vi "Laser 1 TL UI handler L3.vi"(5 "VISA Resource":T2[](array[typedef]), 6 "Numeric":dbl[](array[numeric]), 7 "FP Ops":T4(ring), 8 "Error in":errorcluster caption="Error in (no error)", 9 "Boolean":bool, 10 "I/p string(s)":string[](array[string]), 11 "UI elements cluster":T1) -> (0 "Error out":errorcluster, 3 "Ls1 User Controls 2":T3)   [LabVIEW 2020]
uses:
  Type Defs/Ls1 User Controls.ctl
  Serial Comms/Visa resource.ctl
  Typedefs/Plane Mode.ctl
  Typedefs/Laser control knob.ctl
  Typedefs/PMT control knob.ctl
  Typedefs/XY Stage_Move.ctl
  Typedefs/Frame Size.ctl
  Typedefs/UI ctrl refs cluster.ctl
  Typedefs/test_fpga_control.ctl
  User Interface/Misc/Biology Information.ctl
  User Interface/Misc/Experiment Type.ctl
  Acquisition/Typedefs/Ref DAQ Param.ctl
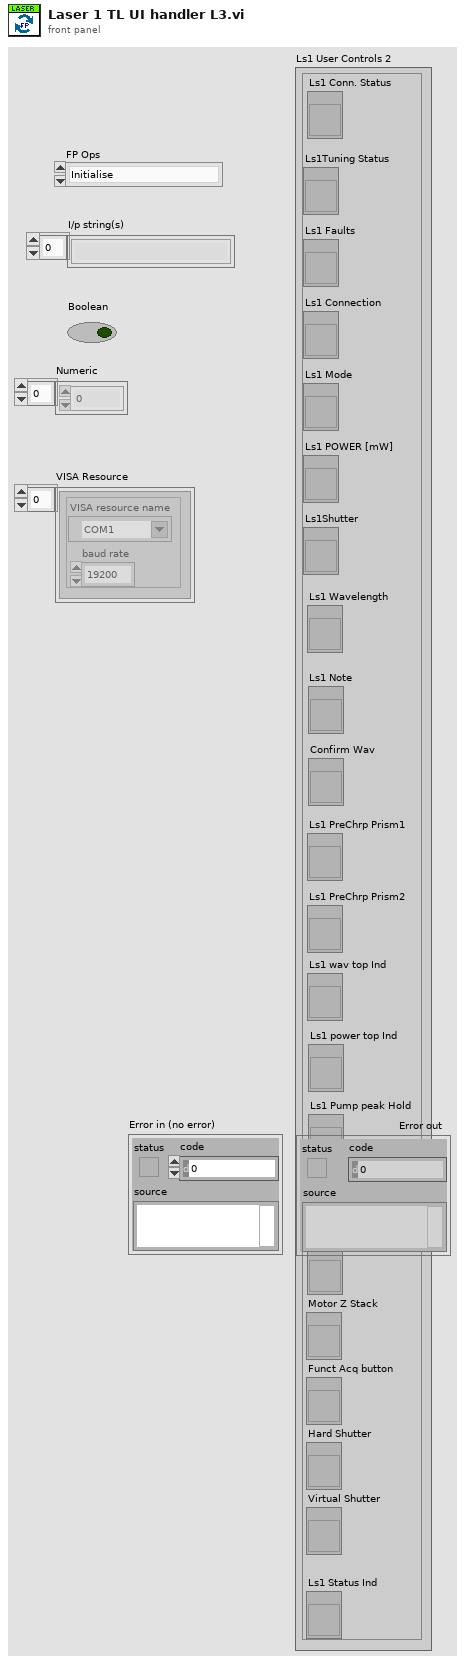
[diagram p1: front panel]
types:
  T1 = typedef "UI ctrl refs cluster.ctl" = cluster{"Top level VI path":path, "Top level VI ref":refnum<vi>, "User menu ref":refnum<k9>, "Sub Panel control":refnum<vi>, "Imaging Param Tab":refnum<vi>, "Occurrence-Start drivers":refnum<k4>, "Occurrence-Speed logging initialised":refnum<k4>, "Occurrence-XYZ stage initialised":refnum<k4>, "Exit button":refnum<vi>, "Status ind":refnum<vi>, "Set as origin":refnum<vi>, "Speed Logging":refnum<vi>, "Time Lapse":refnum<vi>, "Live Imaging":refnum<vi>, "AOL Z Stack":refnum<vi>, "Motor Z Stack":refnum<vi>, "Funct Acq button":refnum<vi>, "Hard Shutter":refnum<vi>, "Virtual Shutter":refnum<vi>, "Laser Power":refnum<vi>, "AOL Mode":refnum<vi>, "Frame Size":refnum<vi>, "Field of View":refnum<vi>, "Dwell Time":refnum<vi>, "Zoom":refnum<vi>, "AOL Z":refnum<vi>, "Objective":refnum<vi>, "Axis":refnum<vi>, "Paths & Names":refnum<vi>, "Experiment folder path (ind.)":refnum<vi>, "Last State (Ind.)":refnum<vi>, "Averages":refnum<vi>, "Angle (degrees)":refnum<vi>, "X centre":refnum<vi>, "Y centre":refnum<vi>, "Plane Mode":refnum<vi>, "# Planes":refnum<vi>, "Z Start":refnum<vi>, "Z Stop":refnum<vi>, "Z Step":refnum<vi>, "PMT 1":refnum<vi>, "PMT 2":refnum<vi>, "Stage XYZ Position":refnum<vi>, "Pockels@Z Start":refnum<vi>, "Pockels@Z Stop":refnum<vi>, "Obtain Z Start":refnum<vi>, "Obtain Z Stop":refnum<vi>, "Live stim.trig.period":refnum<vi>, "Live stim.trig.enable":refnum<vi>, "Movement Correction":refnum<vi>, "Load Reference Image":refnum<vi>, "XY Stage Move":refnum<vi>, "MovCor Cluster":refnum<vi>, "RefDAQParam":refnum<vi>, "Funct. Acq. Pockels Modulation":refnum<vi>, "Ref Laser Power":refnum<vi>, "Enable Video Recording":refnum<vi>, "Video Record-Live Imaging":refnum<vi>, "Video Record-Funct acq":refnum<vi>, "Reference Source":refnum<vi>, "AOL Z-stack Chirps Ready (ind)":refnum<vi>, "Target time between mov.cor. ref triggers (ms)":refnum<vi>, "Funct. Acq. Ref frame save":refnum<vi>, "Tracking button":refnum<vi>, "Show ref plots window":refnum<vi>, "Center freq ind (nm)":refnum<vi>, "Pickup mode (ind)":refnum<vi>, "Logging queue (ind)":refnum<vi>, "Back aperture power (ind.)":refnum<vi>, "Power after objective (ind.)":refnum<vi>, "Switch user":refnum<vi>, "Ls1 Conn. Status":refnum<vi>, "Ls1Tuning Status":refnum<vi>, "Ls1 Faults":refnum<vi>, "Ls1 Connection":refnum<vi>, "Ls1 Mode":refnum<vi>, "Ls1 POWER [mW]":refnum<vi>, "Ls1Shutter":refnum<vi>, "Ls1 Wavelength":refnum<vi>, "Ls1 Note":refnum<vi>, "Ls1 Confirm Wav":refnum<vi>, "Ls1 PreChrp Prism1":refnum<vi>, "Ls1 PreChrp Prism2":refnum<vi>, "Ls1 wav top Ind":refnum<vi>, "Ls1 power top Ind":refnum<vi>, "Ls1 Pump peak Hold":refnum<vi>, "Ls1 Status Ind":refnum<vi>, "Ls1 wav cancel":refnum<vi>, "Experiment Type":refnum<vi>, "Biology Information":refnum<vi>, "Camera recording status":refnum<vi>}
  T2 = typedef "Visa resource.ctl" = cluster{"VISA resource name":refnum<visa-resource-name>, "baud rate":u32}
  T3 = typedef "Ls1 User Controls.ctl" = cluster{"Ls1 Conn. Status":refnum<vi>, "Ls1Tuning Status":refnum<vi>, "Ls1 Faults":refnum<vi>, "Ls1 Connection":refnum<vi>, "Ls1 Mode":refnum<vi>, "Ls1 POWER [mW]":refnum<vi>, "Ls1Shutter":refnum<vi>, "Ls1 Wavelength":refnum<vi>, "Ls1 Note":refnum<vi>, "Confirm Wav":refnum<vi>, "Ls1 PreChrp Prism1":refnum<vi>, "Ls1 PreChrp Prism2":refnum<vi>, "Ls1 wav top Ind":refnum<vi>, "Ls1 power top Ind":refnum<vi>, "Ls1 Pump peak Hold":refnum<vi>, "Live Imaging":refnum<vi>, "AOL Z Stack":refnum<vi>, "Motor Z Stack":refnum<vi>, "Funct Acq button":refnum<vi>, "Hard Shutter":refnum<vi>, "Virtual Shutter":refnum<vi>, "Ls1 Status Ind":refnum<vi>}
  T4 = enum16{"Initialise", "Disable Controls", "Enable Controls", "Update Connection Info", "Update Laser Warning", "Update Laser status", "Update Laser Wav.", "Update prechiper settings", "Update Laser Note", "Update Shutter Status"}
  T5 = enum8{"Enabled", "Disabled", "Disabled and Grayed Out"}
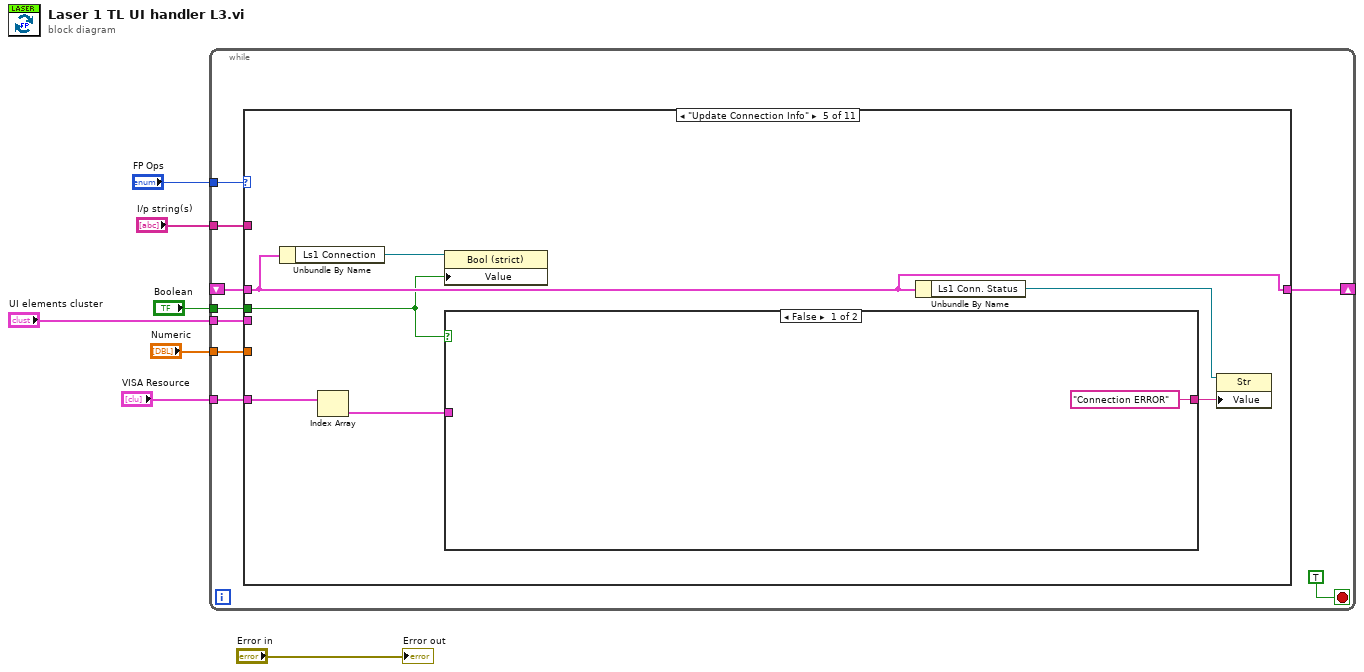
[diagram p0: block diagram]
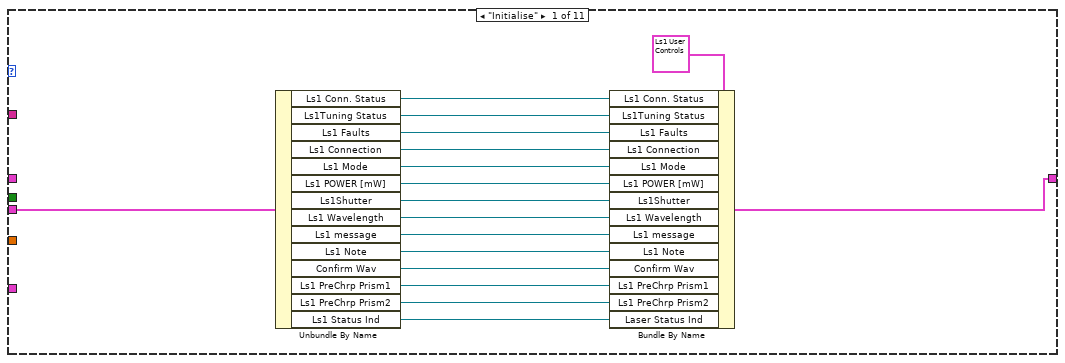
[diagram p2: hidden frame]
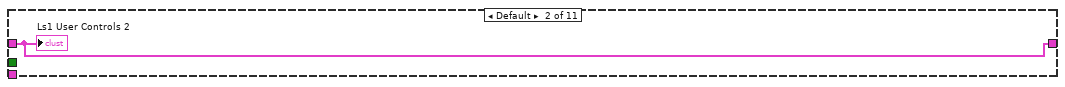
[diagram p3: hidden frame]
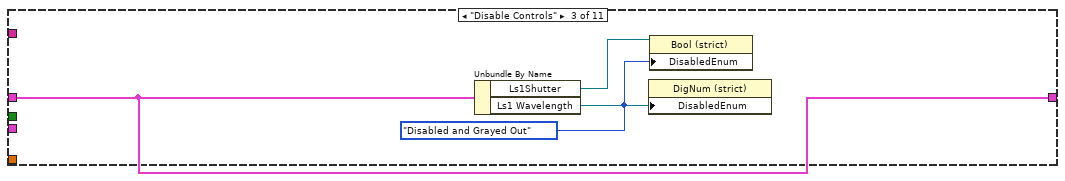
[diagram p4: hidden frame]
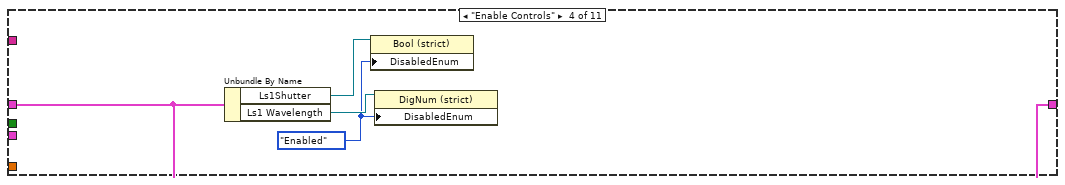
[diagram p5: hidden frame]
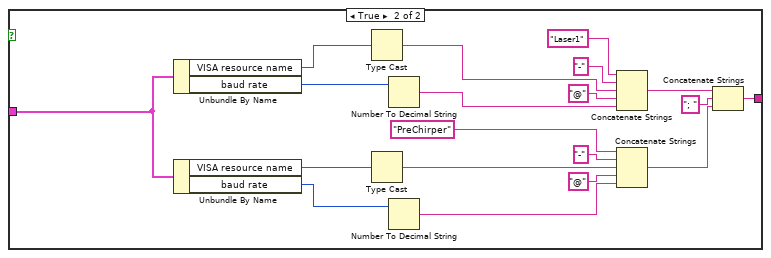
[diagram p6: hidden frame]
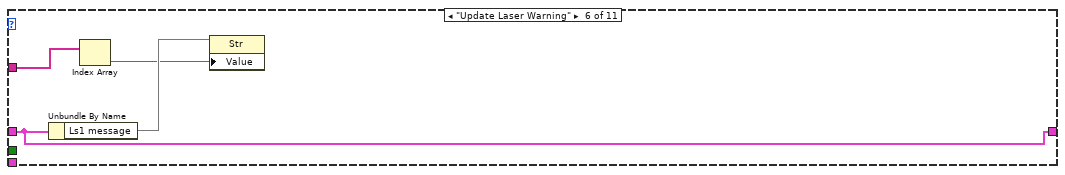
[diagram p7: hidden frame]
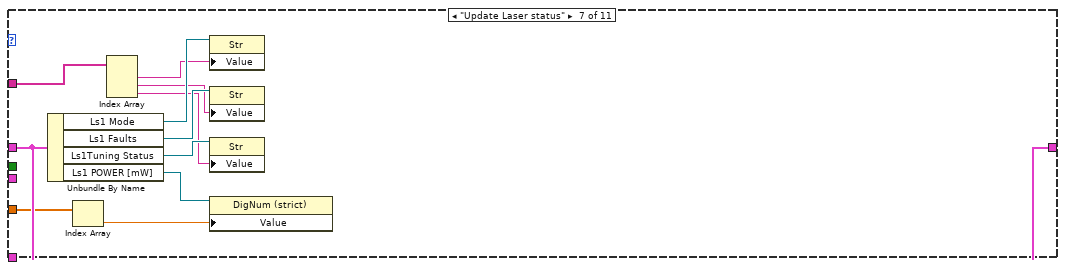
[diagram p8: hidden frame]
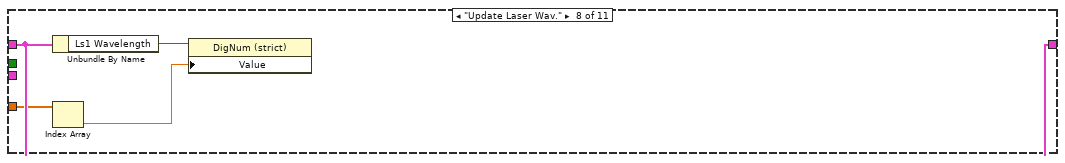
[diagram p9: hidden frame]
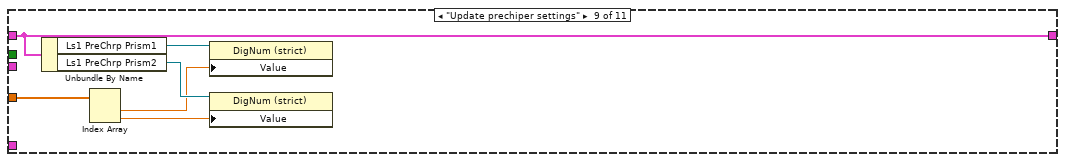
[diagram p10: hidden frame]
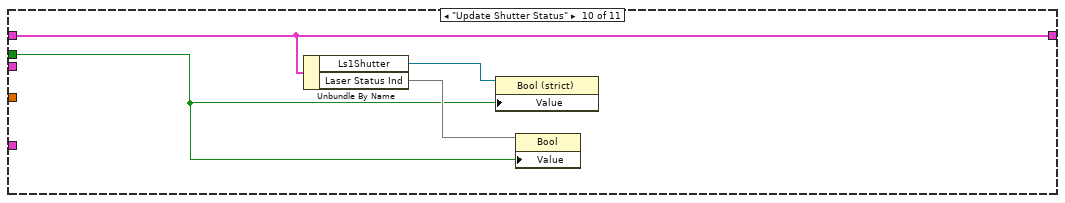
[diagram p11: hidden frame]
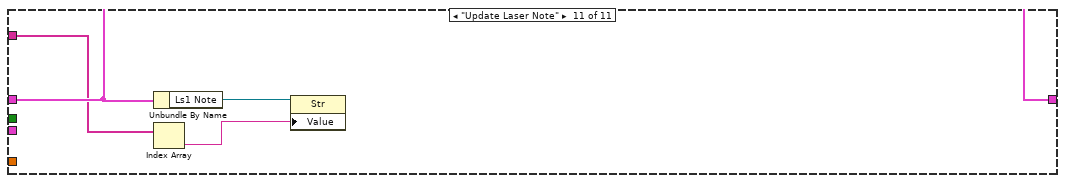
[diagram p12: hidden frame]
diagram:
  n1 = while {
    tunnel: "FP Ops" -> [w16]
    tunnel: "Boolean" -> [w14]
    tunnel: "I/p string(s)" -> [w13]
    tunnel: "VISA Resource" -> [w12]
    tunnel: "Numeric" -> [w11]
    shift-right: [w8] -> _
    shift-left: _ -> [w15]
    tunnel: "UI elements cluster" -> [w9]
    stop <- TRUE stop-if-true
    n2 = case shown="\"Update Connection Info\"" w16 {
      tunnel: w15 -> [_ w34 w35 w39 w48 w73 w84 w88 w94 w97 w102]
      tunnel: w13 -> [_ _ _ _ _ w71 w79 _ _ _ w100]
      tunnel: w14 -> [_ _ _ _ w43 _ _ _ _ w95 _]
      tunnel: w11 -> [_ _ _ _ _ _ w75 w85 w91 _ _]
      tunnel: w12 -> [_ _ _ _ w45 _ _ _ _ _ _]
      tunnel: w9 -> [w19 _ _ _ _ _ _ _ _ _ _]
      tunnel: [w18 w34 w35 w39 w48 w73 w84 w88 w94 w97 w102] -> w8
      frame "Initialise" {
        n3 = Unbundle By Name(w19) -> ("Ls1 Conn. Status"=w32:refnum<vi>, "Ls1Tuning Status"=w31:refnum<vi>, "Ls1 Faults"=w30:refnum<vi>, "Ls1 Connection"=w29:refnum<vi>, "Ls1 Mode"=w28:refnum<vi>, "Ls1 POWER [mW]"=w27:refnum<vi>, "Ls1Shutter"=w26:refnum<vi>, "Ls1 Wavelength"=w25:refnum<vi>, "Ls1 message"=w24:refnum<vi>, "Ls1 Note"=w23:refnum<vi>, "Confirm Wav"=w22:refnum<vi>, "Ls1 PreChrp Prism1"=w21:refnum<vi>, "Ls1 PreChrp Prism2"=w20:refnum<vi>, "Ls1 Status Ind"=w17:refnum<vi>)
        n4 = Bundle By Name(cluster=T3 {"Ls1 Conn. Status"=refnum, "Ls1Tuning Status"=refnum, "Ls1 Faults"=refnum, "Ls1 Connection"=refnum, "Ls1 Mode"=refnum, "Ls1 POWER [mW]"=refnum, "Ls1Shutter"=refnum, "Ls1 Wavelength"=refnum, "Ls1 Note"=refnum, "Confirm Wav"=refnum, "Ls1 PreChrp Prism1"=refnum, "Ls1 PreChrp Prism2"=refnum, "Ls1 wav top Ind"=refnum, "Ls1 power top Ind"=refnum, "Ls1 Pump peak Hold"=refnum, "Live Imaging"=refnum, "AOL Z Stack"=refnum, "Motor Z Stack"=refnum, "Funct Acq button"=refnum, "Hard Shutter"=refnum, "Virtual Shutter"=refnum, "Ls1 Status Ind"=refnum} ("Ls1 User Controls"), "Ls1 Conn. Status"=w32, "Ls1Tuning Status"=w31, "Ls1 Faults"=w30, "Ls1 Connection"=w29, "Ls1 Mode"=w28, "Ls1 POWER [mW]"=w27, "Ls1Shutter"=w26, "Ls1 Wavelength"=w25, "Ls1 message"=w24, "Ls1 Note"=w23, "Confirm Wav"=w22, "Ls1 PreChrp Prism1"=w21, "Ls1 PreChrp Prism2"=w20, "Laser Status Ind"=w17) -> (w18:T3)
      }
      frame Default {
        "Ls1 User Controls 2" <- w34
      }
      frame "Disable Controls" {
        w36 = T5."Disabled and Grayed Out" ("Disabled")
        n5 = Unbundle By Name(w35) -> ("Ls1Shutter"=w38:refnum<vi>, "Ls1 Wavelength"=w37:refnum<vi>)
        n6 = property class="DigNum (strict)"(reference=w37, "DisabledEnum"=w36) -> ()  [unwired: 1 in, 2 out]
        n7 = property class="Bool (strict)"(reference=w38, "DisabledEnum"=w36) -> ()  [unwired: 1 in, 2 out]
      }
      frame "Enable Controls" {
        w40 = T5."Enabled" ("Disabled")
        n8 = Unbundle By Name(w39) -> ("Ls1Shutter"=w42:refnum<vi>, "Ls1 Wavelength"=w41:refnum<vi>)
        n9 = property class="Bool (strict)"(reference=w42, "DisabledEnum"=w40) -> ()  [unwired: 1 in, 2 out]
        n10 = property class="DigNum (strict)"(reference=w41, "DisabledEnum"=w40) -> ()  [unwired: 1 in, 2 out]
      }
      frame "Update Connection Info" {
        n11 = Unbundle By Name(w48) -> ("Ls1 Connection"=w47:refnum<vi>)
        n12 = Index Array(array=w45) -> (element=w46:T2)  [unwired: 1 in]
        n13 = property class="Bool (strict)"(reference=w47, "Value"=w43) -> ()  [unwired: 1 in, 2 out]
        n14 = case shown="False" w43 {
          tunnel: w46 -> [_ w52]
          tunnel: ["Connection ERROR" w51] -> w44
          frame False {
          }
          frame True {
            n15 = Unbundle By Name(w52) -> ("VISA resource name"=w69:refnum<visa-resource-name>, "baud rate"=w68:u32)
            n16 = Unbundle By Name(w52) -> ("VISA resource name"=w57:refnum<visa-resource-name>, "baud rate"=w53:u32)
            n17 = Type Cast(x=w69) -> (*(type *) &x=w64:string)  [unwired: 1 in]
            n18 = Type Cast(x=w57) -> (*(type *) &x=w59:string)  [unwired: 1 in]
            n19 = Number To Decimal String(number=w68) -> (decimal integer string=w63:string)  [unwired: 1 in]
            n20 = Number To Decimal String(number=w53) -> (decimal integer string=w58:string)  [unwired: 1 in]
            n21 = Concatenate Strings("Laser1", "-" ("string"), w64, "@" ("string"), w63) -> (w56:string)
            n22 = Concatenate Strings("PreChirper", "-" ("string"), w59, "@" ("string"), w58) -> (w55:string)
            n23 = Concatenate Strings(w56, "; ", w55) -> (w51:string)
          }
        }
        n24 = Unbundle By Name(w48) -> ("Ls1 Conn. Status"=w49:refnum<vi>)
        n25 = property class="Str"(reference=w49, "Value"=w44) -> ()  [unwired: 1 in, 2 out]
      }
      frame "Update Laser Warning" {
        n26 = Unbundle By Name(w73) -> ("Ls1 message"=w72)
        n27 = Index Array(array=w71) -> (element=w70:string)  [unwired: 1 in]
        n28 = property class="Str"(reference=w72, "Value"=w70) -> ()  [unwired: 1 in, 2 out]
      }
      frame "Update Laser status" {
        n29 = Unbundle By Name(w84) -> ("Ls1 Mode"=w83:refnum<vi>, "Ls1 Faults"=w82:refnum<vi>, "Ls1Tuning Status"=w81:refnum<vi>, "Ls1 POWER [mW]"=w80:refnum<vi>)
        n30 = Index Array(array=w75) -> (element=w74:dbl)  [unwired: 1 in]
        n31 = Index Array(array=w79) -> (element #1=w78:string, element #2=w77:string, element #3=w76:string)  [unwired: 3 in]
        n32 = property class="Str"(reference=w83, "Value"=w78) -> ()  [unwired: 1 in, 2 out]
        n33 = property class="Str"(reference=w82, "Value"=w77) -> ()  [unwired: 1 in, 2 out]
        n34 = property class="Str"(reference=w81, "Value"=w76) -> ()  [unwired: 1 in, 2 out]
        n35 = property class="DigNum (strict)"(reference=w80, "Value"=w74) -> ()  [unwired: 1 in, 2 out]
      }
      frame "Update Laser Wav." {
        n36 = Unbundle By Name(w88) -> ("Ls1 Wavelength"=w87:refnum<vi>)
        n37 = Index Array(array=w85) -> (element=w86:dbl)  [unwired: 1 in]
        n38 = property class="DigNum (strict)"(reference=w87, "Value"=w86) -> ()  [unwired: 1 in, 2 out]
      }
      frame "Update prechiper settings" {
        n39 = Unbundle By Name(w94) -> ("Ls1 PreChrp Prism1"=w93:refnum<vi>, "Ls1 PreChrp Prism2"=w92:refnum<vi>)
        n40 = Index Array(array=w91) -> (element #1=w90:dbl, element #2=w89:dbl)  [unwired: 2 in]
        n41 = property class="DigNum (strict)"(reference=w93, "Value"=w90) -> ()  [unwired: 1 in, 2 out]
        n42 = property class="DigNum (strict)"(reference=w92, "Value"=w89) -> ()  [unwired: 1 in, 2 out]
      }
      frame "Update Shutter Status" {
        n43 = Unbundle By Name(w97) -> ("Ls1Shutter"=w98:refnum<vi>, "Laser Status Ind"=w96)
        n44 = property class="Bool (strict)"(reference=w98, "Value"=w95) -> ()  [unwired: 1 in, 2 out]
        n45 = property class="Bool"(reference=w96, "Value"=w95) -> ()  [unwired: 1 in, 2 out]
      }
      frame "Update Laser Note" {
        n46 = Unbundle By Name(w102) -> ("Ls1 Note"=w101:refnum<vi>)
        n47 = Index Array(array=w100) -> (element=w99:string)  [unwired: 1 in]
        n48 = property class="Str"(reference=w101, "Value"=w99) -> ()  [unwired: 1 in, 2 out]
      }
    }
  }
  "Error out" <- "Error in"
